vi "Open Report File.vi"(8 "error in (no error)":errorcluster, 10 "Path":path, 11 "Text Report In":refnum<class "Text Report.lvclass">) -> (0 "error out":errorcluster, 3 "Text Report Out":refnum<class "Text Report.lvclass">)   [LabVIEW 2020, in "Reports.lvlib" / "Text Report.lvclass"]
uses:
  Text Report.lvclass
  Text Report.lvclass/Text Report.ctl
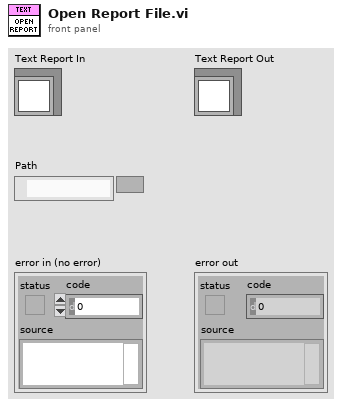
[diagram p1: front panel]
types:
  T1 = enum16{"open", "replace", "create", "open or create", "replace or create", "replace or create with confirmation"}
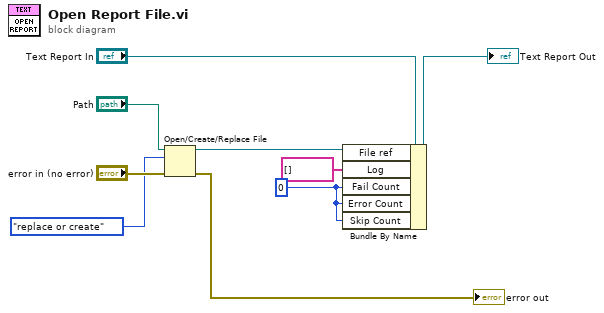
[diagram p0: block diagram]
diagram:
  w1 = 0 ("Fail Count")
  n1 = Open/Create/Replace File(file path (use dialog)="Path", error in="error in (no error)", operation (0:open)=T1."replace or create") -> (refnum out=w3:refnum<file>, error out=→"error out":errorcluster)  [unwired: 3 in, 1 out]
  n2 = Bundle By Name(cluster="Text Report In", "File ref"=w3, "Log"=string[] [], "Fail Count"=w1, "Error Count"=w1, "Skip Count"=w1) -> (→"Text Report Out":refnum<class "Text Report.lvclass">)
